vi "TCP Read Length and Value (Array I16).vi"(8 "error in (no error)":errorcluster, 10 "timeout ms (1000)":i32=1000, 11 "TCP Network Connection in":refnum<k5>) -> (0 "error out":errorcluster, 2 "Output":i16[](array[numeric]), 3 "TCP Network Connection out":refnum<k5>)   [LabVIEW 2024]
doc: "This software is licensed for use under the “MIT License\"\nCopyright (c) 2019 Scott Hannahs, sth@alum.mit.edu\n\nPermission is hereby granted, free of charge, to any person obtaining a copy of this software and associated documentation files (the \"Software\"), to deal in the Software without restriction, including without limitation the rights to use, copy, modify, merge, publish, distribute, sublicense, and/or sell copies of the Software, and to permit persons to whom the Software is furnished to do so, subject to the following conditions: The above copyright notice and this permission notice shall be included in all copies or substantial portions of the Software.\n\nTHE SOFTWARE IS PROVIDED \"AS IS\", WITHOUT WARRANTY OF ANY KIND, EXPRESS OR IMPLIED, INCLUDING BUT NOT LIMITED TO THE WARRANTIES OF MERCHANTABILITY, FITNESS FOR A PARTICULAR PURPOSE AND NONINFRINGEMENT. IN NO EVENT SHALL THE AUTHORS OR COPYRIGHT HOLDERS BE LIABLE FOR ANY CLAIM, DAMAGES OR OTHER LIABILITY, WHETHER IN AN ACTION OF CONTRACT, TORT OR OTHERWISE, ARISING FROM, OUT OF OR IN CONNECTION WITH THE SOFTWARE OR THE USE OR OTHER DEALINGS IN THE SOFTWARE."
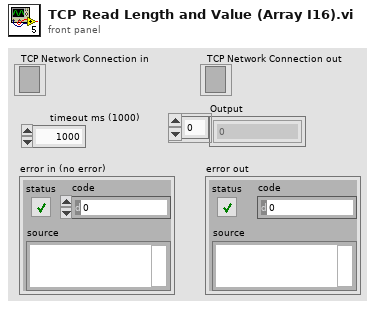
[diagram p1: front panel]
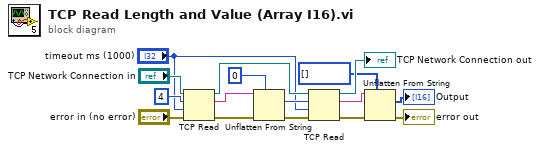
[diagram p0: block diagram]
diagram:
  n1 = TCP Read(connection ID="TCP Network Connection in", bytes to read=4, error in (no error)="error in (no error)", 9:"timeout ms (1000)") -> (connection ID out=w10:refnum<k5>, data out=w8:string, error out=w5:errorcluster)  [unwired: 1 in]
  n2 = Unflatten From String(type=u32 0 ("bytes to read"), binary string=w8, error in (no error)=w5) -> (value=w6:u32, error out=w3:errorcluster)  [unwired: 2 in, 1 out]
  n3 = TCP Read(connection ID=w10, bytes to read=w6, error in (no error)=w3, 9:"timeout ms (1000)") -> (connection ID out=→"TCP Network Connection out":refnum<k5>, data out=w15:string, error out=w13:errorcluster)  [unwired: 1 in]
  n4 = Unflatten From String(type=i16[] [], binary string=w15, error in (no error)=w13) -> (value=→"Output":i16[], error out=→"error out":errorcluster)  [unwired: 2 in, 1 out]
